vi "Remove empty impulses.vi"(1 "Data out":dbl[][](array[numeric])) -> (0 "Data out 2":dbl[][](array[numeric]))   [LabVIEW 2013, in "Impulse Data.lvclass"]
uses:
  Impulse Data.lvclass
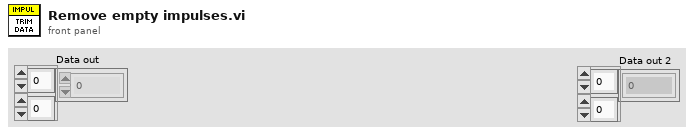
[diagram p1: front panel]
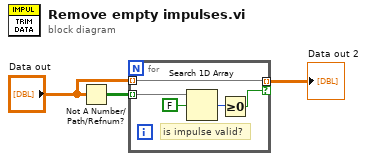
[diagram p0: block diagram]
diagram:
  n1 = Not A Number/Path/Refnum?(number/path/refnum="Data out") -> (NaN/Path/Refnum?=w3:bool[][])
  n2 = for {
    tunnel: w3 -> [w8] mode=indexing
    tunnel: [w6] -> w1 mode=indexing if=w4
    tunnel: "Data out" -> [w6] mode=indexing
    # "is impulse valid?"
    n3 = Search 1D Array(1D array=w8, element=FALSE) -> (index of element=w5:i32)  [unwired: 1 in]
    n4 = Greater Or Equal To 0?(x=w5) -> (x >= 0?=w4:bool)
  }
  "Data out 2" <- w1
